vi "发送Task B任务.vi"(7 "消息优先级（标准）":T1=enum."Normal", 8 "error in (no error)":cluster{"状态":bool, "代码":i32, "源":string} caption="错误输入（无错误）", 10 "数据":i32, 11 "消息待入队列":refnum<class "Message Enqueuer.lvclass">) -> (0 "error out":cluster{"状态":bool, "代码":i32, "源":string} caption="错误输出")   [LabVIEW 2013, in "Task B操作者.lvlib" / "Task B任务消息.lvclass"]
uses:
  <vilib>/ActorFramework/Message Enqueuer/Message Enqueuer.lvclass
  <vilib>/ActorFramework/Message Enqueuer/Message Priority.ctl
  <vilib>/ActorFramework/Message Enqueuer/Message Enqueuer.lvclass/Message Enqueuer.ctl
  <vilib>/ActorFramework/Message Priority Queue/Priority Enqueue.vi
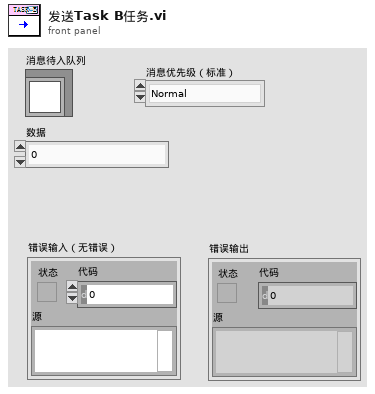
[diagram p1: front panel]
types:
  T1 = typedef "Actor Framework.lvlib/Message Enqueuer.lvclass/Message Priority.ctl" = enum16{"Low", "Normal", "High"}
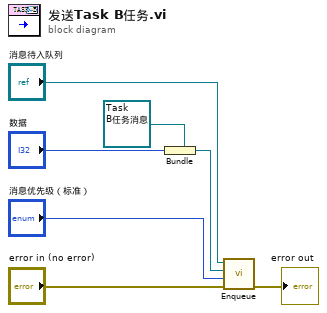
[diagram p0: block diagram]
diagram:
  n1 = Bundle(cluster=refnum<class "Task B任务消息.lvclass"> refnum ("Object"), "数据") -> (w3:refnum<class "Task B任务消息.lvclass">)
  n2 = call <vilib>:"Enqueue.vi"("error in (no error)"="error in (no error)", "Message Priority (Normal)"="消息优先级（标准）", "Message"=w3, "Message Enqueuer in"="消息待入队列") -> ("error out"=→"error out":errorcluster)  [unwired: 6 in, 1 out]
